vi "Blueboard_ADC_v1.vi"(8 "error in (no error)":errorcluster, 9 "Message IN":string, 10 "Blue Board Enum":T1=enum."TEST_POINT", 11 "ControlBoard VISA":refnum<visa-resource-name>="ControlBoard") -> (0 "error out":errorcluster, 1 "Message OUT":string, 2 "VISA Refnum out":refnum<visa-resource-name>, 3 "Result":dbl)   [LabVIEW 2019]
uses:
  Ctls/ADC_Select_v1.ctl
  <vilib>/Instr/_visa.llb/VISA Flush IO Buffer Mask.ctl
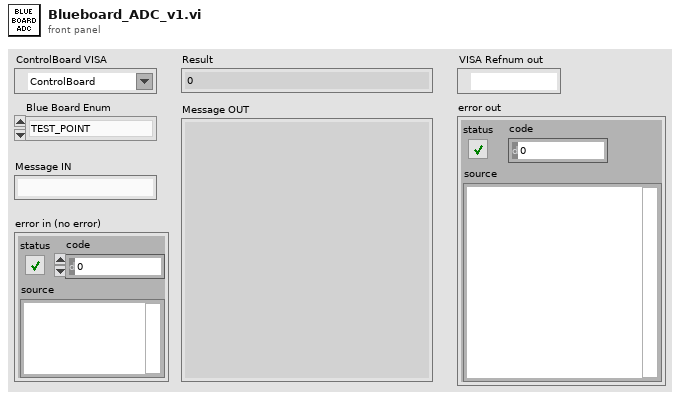
[diagram p1: front panel]
types:
  T1 = typedef "ADC_Select_v1.ctl" = enum16{"INVA_ISENSE_U", "INVA_ISENSE_V", "INVA_ISENSE_W", "INVA_UDC", "INVA_TEMP", "HB_TEMP", "AUXB_TEMP", "VLINE_AB", "VLINE_BC", "VLINE_CA", "VSENSE_POS_24V", "VSENSE_POS_5V", "VSENSE_NEG_15V", "INVB_ISENSE_U", "INV_B_ISENSEV", "INVB_ISENSE_W", "INVB_UDC", "INVB_TEMP", "AUXA_TEMP", "AUXC_TEMP", "VOUT_AB", "VOUT_BC", "VOUT_CA", "VSENSE_POS_15V", "VSENSE_POS_3P3V", "TEST_POINT"}
  T2 = typedef "VISA Flush IO Buffer Mask.ctl" = u16
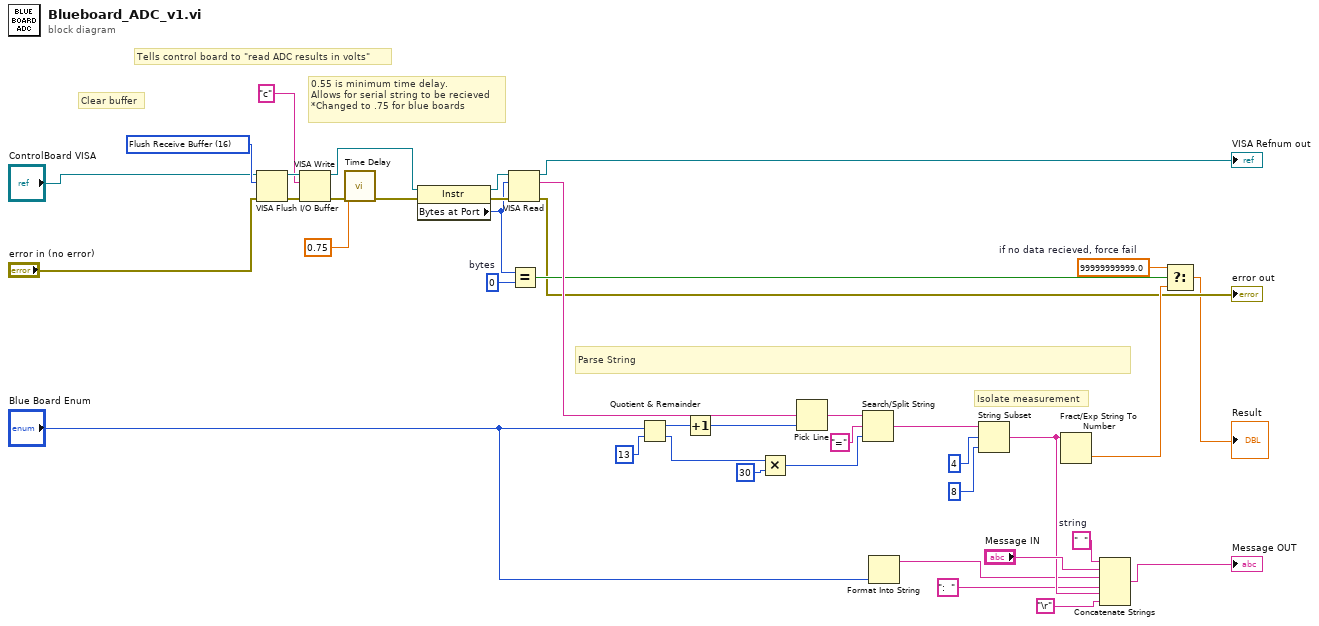
[diagram p0: block diagram]
diagram:
  w10 = "  "  # string
  w16 = 99999999999.0  # if no data recieved, force fail
  w19 = u32 0  # bytes
  w24 = T2 16 items=["Flush Receive Buffer"=16, "Write Transmit Buffer to Device"=32, "Flush Receive Buffer (No I/O)"=64, "Flush Transmit Buffer"=128] ("Mask")
  # "Isolate measurement"
  # "Clear buffer"
  # "Parse String"
  # "0.55 is minimum time delay.\nAllows for serial string to be recieved\n*Changed to .75 for blue boards"
  # "Tells control board to \"read ADC results in volts\""
  n1 = VISA Flush I/O Buffer(VISA resource name="ControlBoard VISA", mask (16)=w24, error in (no error)="error in (no error)") -> (VISA resource name out=w26:refnum<visa-resource-name>, error out=w27:errorcluster)
  n2 = VISA Write(VISA resource name=w26, write buffer="c", error in (no error)=w27) -> (VISA resource name out=w29:refnum<visa-resource-name>, error out=w25:errorcluster)  [unwired: 1 out]
  n3 = call "Time Delay"("error in (no error)"=w25, "Delay Time (s)"=0.75) -> ("error out"=w28:errorcluster)  [unwired: 9 in]
  n4 = property class="Instr"(reference=w29, error in=w28) -> (reference out=w22:refnum<visa-resource-name>, error out=w23:errorcluster, "Bytes at Port"=w20:u32)
  n5 = VISA Read(VISA resource name=w22, byte count=w20, error in (no error)=w23) -> (VISA resource name out=→"VISA Refnum out":refnum<visa-resource-name>, read buffer=w38:string, error out=→"error out":errorcluster)  [unwired: 1 out]
  n6 = Equal?(x=w20, y=w19) -> (x = y?=w17:bool)
  n7 = Quotient & Remainder(x="Blue Board Enum", y=13) -> (x-y*floor(x/y)=w33:i32, floor(x/y)=w35:i32)
  n8 = Increment(x=w33) -> (x+1=w34:i32)
  n9 = Multiply(x=w35, y=30) -> (x*y=w37:i32)
  n10 = Pick Line(multi-line string=w38, line index=w34) -> (output string=w39:string)  [unwired: 1 in]
  n11 = Search/Split String(string=w39, search string/char (-)="=" ("regular expression"), offset (0)=w37) -> (match + rest of string=w31:string)  [unwired: 2 out]
  n12 = Format Into String("Blue Board Enum") -> (resulting string=w2:string)  [unwired: 3 in, 1 out]
  n13 = String Subset(string=w31, offset (0)=4, length (rest)=8 ("offset (0)")) -> (substring=w12:string)
  n14 = Fract/Exp String To Number(string=w12) -> (number=w18:dbl)  [unwired: 3 in, 1 out]
  n15 = Concatenate Strings(w10, "Message IN", w2, ":  ", w12, "\r") -> (→"Message OUT":string)
  n16 = Select(t=w16, s=w17, f=w18) -> (s? t:f=→"Result":dbl)
